vi "Example-血氧仪.vi"() -> ()   [LabVIEW 2018]
uses:
  17504645-33d6-4640-8c4b-92a03107a571.vi
  d24536d2-1b2e-48eb-9735-a10c89dc3041.vi
  40ac2d0d-2d52-431a-8f5c-900a3948c8a2.vi
panel:
  in  "Voltage(V)":dbl=3.3 format="%#_13g"
  in  "Frequency(Hz)":i32(ring)=400 items=["1"=1, "10"=10, "40"=40, "100"=100, "400"=400, "1000"=1000, "4000"=4000, "10000"=10000, "40000"=40000, "100000"=100000, "400000"=400000, "1000000"=1000000, "4000000"=4000000, "10000000"=10000000]
  in  "停止":bool
  in  "addr":u8=87 format="%.0x"
  out "数值":i32
  out "波形图表":cluster{u32, u32}(graph)
  out "SerialNumber":string
  out "rxcount out":i32
  out "rgRX":u8[](array[numeric])
  in  "Tx data":u8[][](array[numeric])=[[9, 64], [2, 12], [3, 0], [4, 0], [5, 0], [6, 0], [8, 15], [9, 3], [10, 39], [12, 50], [13, 50], [16, 127]] format="%.0x"
  in  "SDA IO(0~15)":i32=1
  in  "SCL IO(0~15)":i32
  out "returns":i32[](array[numeric])
  out "error out":errorcluster caption="错误输出"
  in  "error in (no error)":errorcluster caption="错误输入（无错误）"
  out "ftHandle out":u64=363562184
  in  "设备索引":i32
  # "72 75"
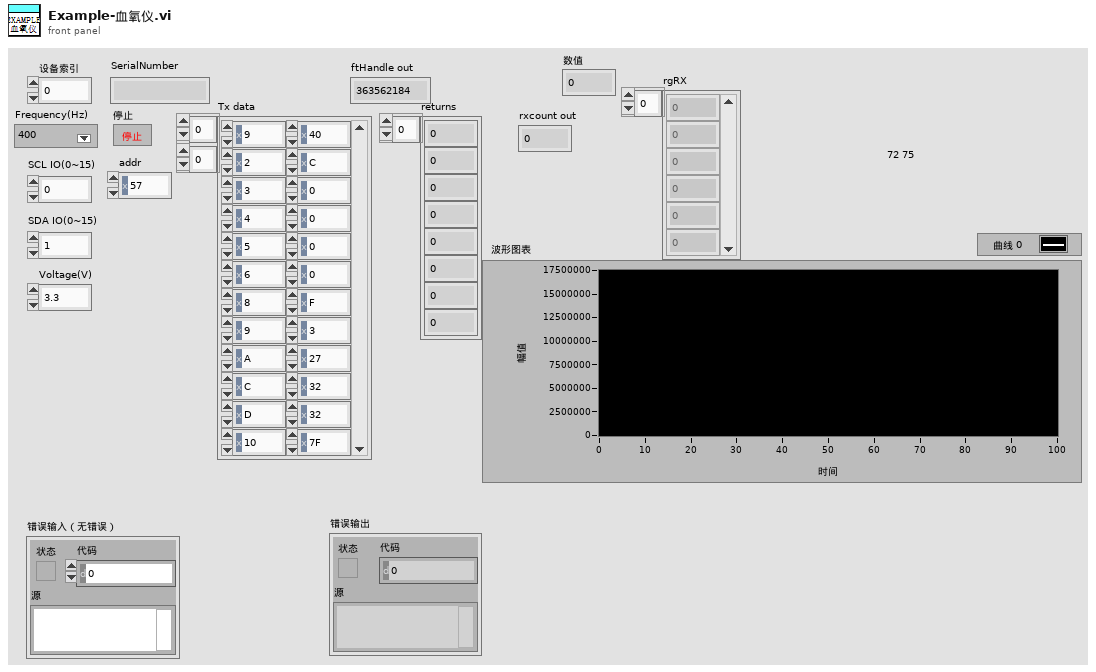
[diagram p1: front panel]
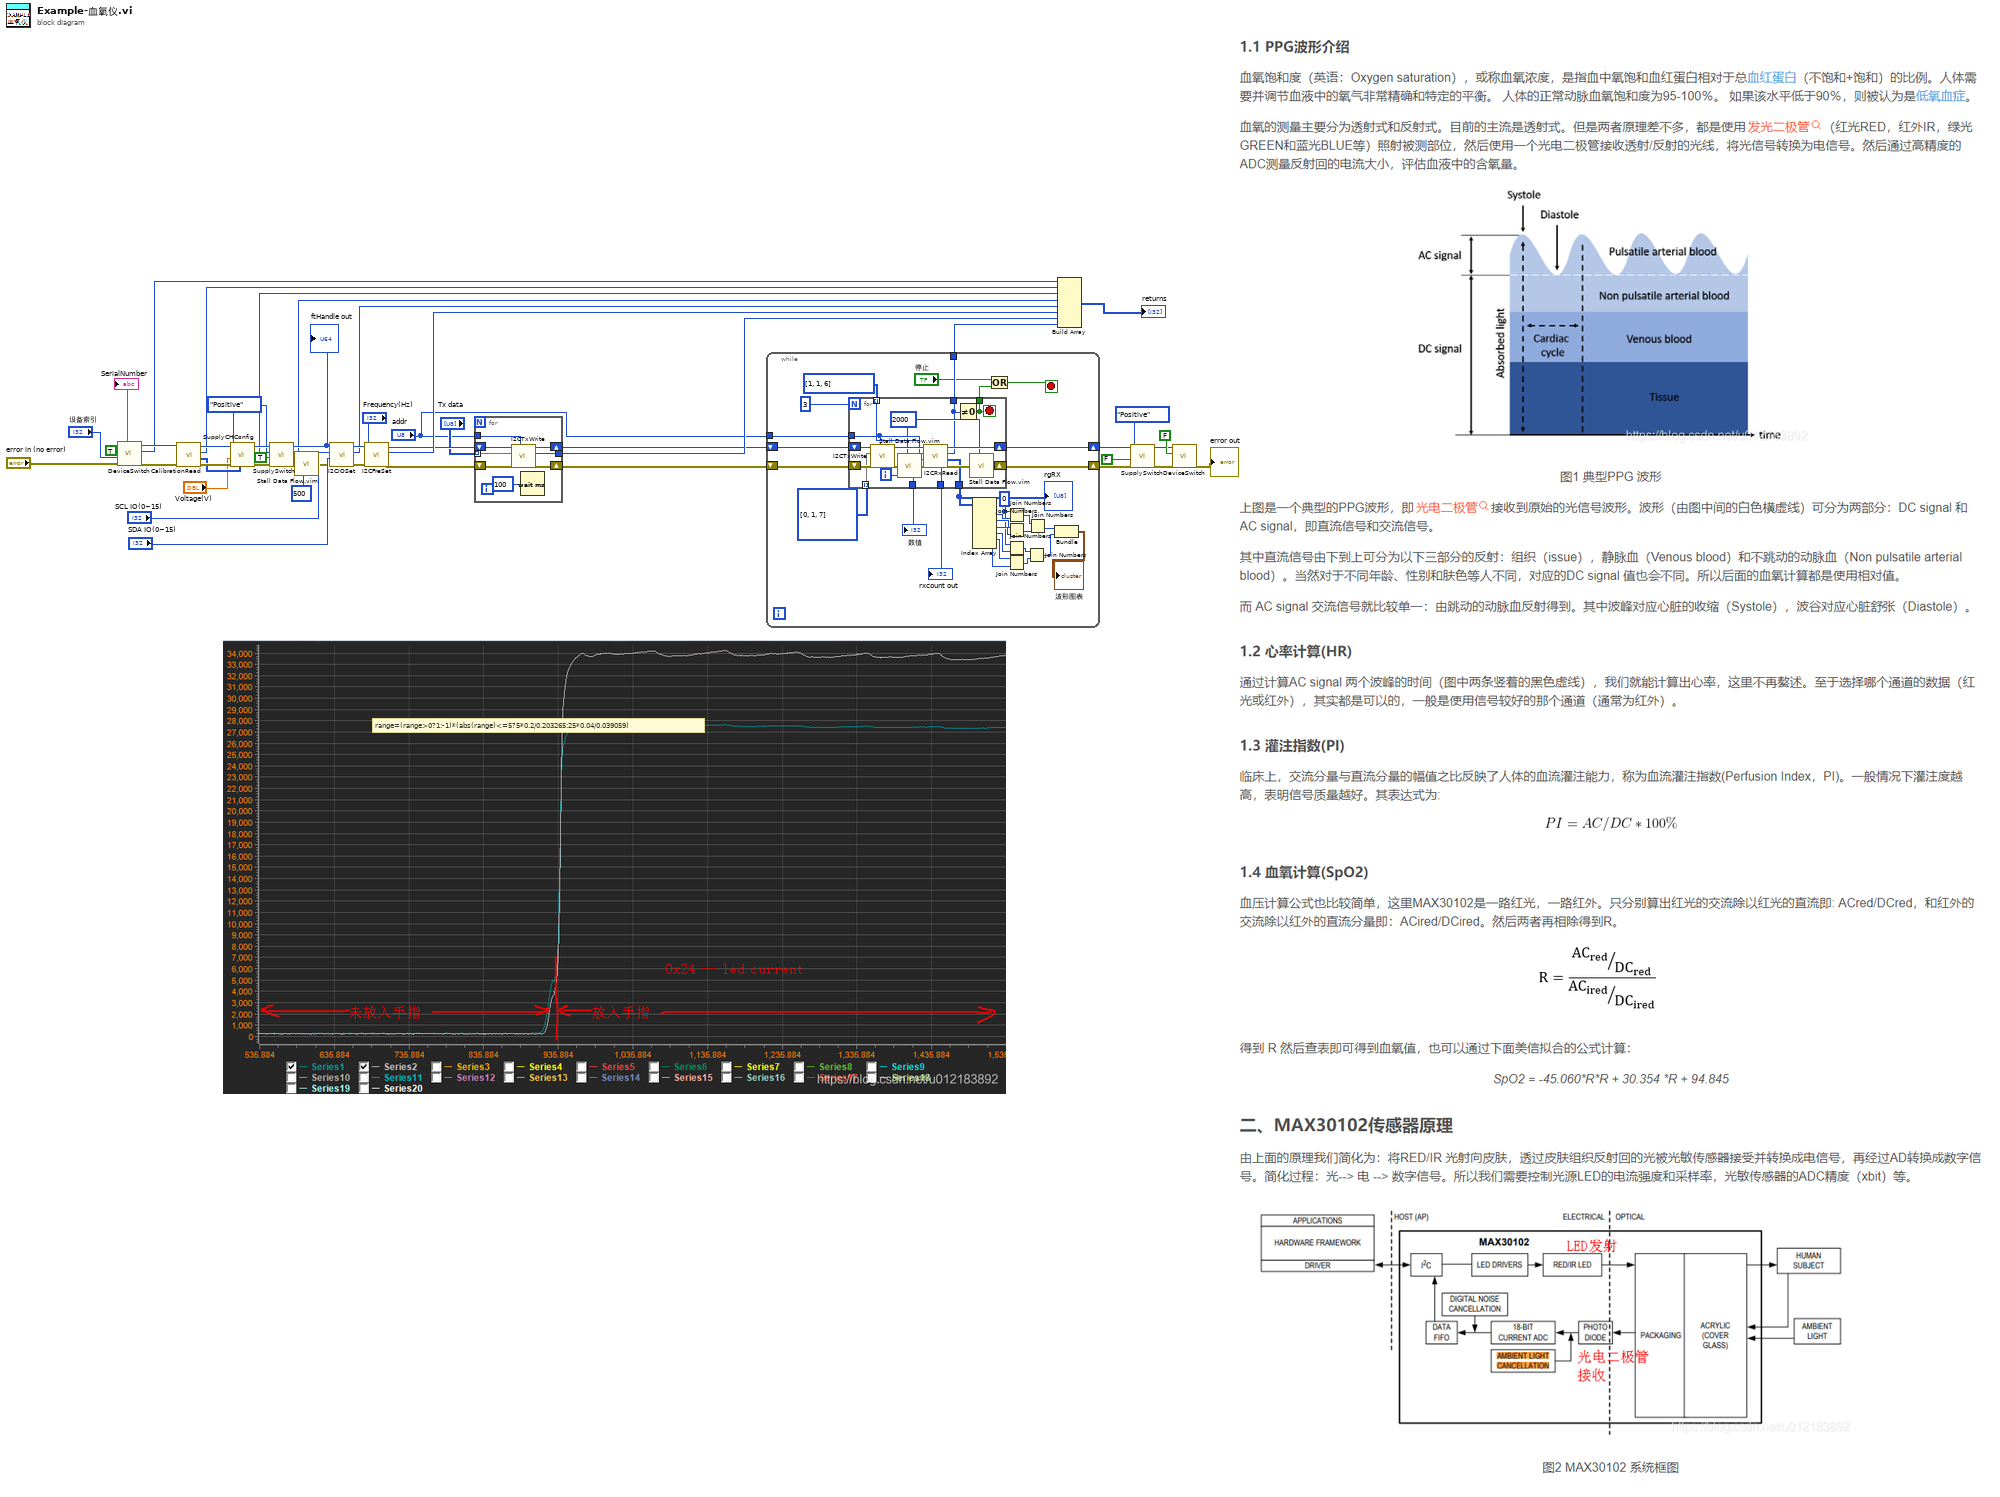
[diagram p0: block diagram]
diagram:
  w24 = enum16{"Positive", "Negative"}."Positive" ("CH")
  # "range=(range>0?1:-1)*(abs(range)<=5?5*0.2/0.203265:25*0.04/0.039059)"
  n1 = call "DeviceSwitch.vi"("error in (no error)"="error in (no error)", "Device Index"="设备索引", "Open"=TRUE) -> ("error out"=w19:errorcluster, "function return"=w15:i32, "handle out"=w18:u64, "SerialNumber"=→"SerialNumber":string)  [unwired: 4 in, 1 out]
  n2 = call "CalibrationRead.vi"("handle"=w18, "error in (no error)"=w19) -> ("handle out"=w21:u64, "function return"=w14:i32, "CalArray"=w20:u8[], "error out"=w22:errorcluster)  [unwired: 5 in]
  n3 = call "SupplyCHConfig.vi"("CalArray"=w20, "error in (no error)"=w22, "Voltage(V)"="Voltage(V)", "CH"=w24, "handle"=w21) -> ("error out"=w25:errorcluster, "function return"=w13:i32, "handle out"=w26:u64)  [unwired: 3 in, 1 out]
  n4 = call "SupplySwitch.vi"("error in (no error)"=w25, "Output"=TRUE, "CH"=w24, "handle"=w26) -> ("error out"=w16:errorcluster, "function return"=w12:i32, "handle out"=w17:u64)  [unwired: 5 in]
  "ftHandle out" <- w17
  n5 = call "Stall Data Flow.vim"("value in"=w16, "milliseconds to wait"=u32 500) -> ("value out"=w4:errorcluster)  [unwired: 1 out]
  n6 = call "I2CIOSet.vi"("error in (no error)"=w4, "SDA IO(0~15)"="SDA IO(0~15)", "SCL IO(0~15)"="SCL IO(0~15)", "handle"=w17) -> ("error out"=w40:errorcluster, "function return"=w36:i32, "handle out"=w37:u64)  [unwired: 5 in]
  n7 = call "I2CFreSet.vi"("error in (no error)"=w40, "Frequency(Hz)"="Frequency(Hz)", "handle"=w37) -> ("error out"=w31:errorcluster, "function return"=w35:i32, "handle out"=w34:u64)  [unwired: 6 in]
  n8 = for {
    tunnel: "Tx data" -> [w48] mode=indexing
    tunnel: [w50] -> w30
    tunnel: "addr" -> [w49]
    shift-right: [w51] -> w2
    shift-left: w34 -> [w54]
    shift-right: [w53] -> w32
    shift-left: w31 -> [w52]
    n9 = call "I2CTxWrite.vi"("addr"=w49, "error in (no error)"=w52, "data"=w48, "handle"=w54) -> ("error out"=w53:errorcluster, "function return"=w50:i32, "handle out"=w51:u64)  [unwired: 5 in]
    n10 = Wait (ms)(milliseconds to wait=u32 100 ("等待时间（毫秒）")) -> ()  [unwired: 1 out]
  }
  n11 = while {
    tunnel: [w79] -> w29
    tunnel: "addr" -> [w75]
    shift-right: [w82] -> w10
    shift-left: w32 -> [w83]
    shift-right: [w81] -> w8
    shift-left: w2 -> [w80]
    stop <- w65 stop-if-true
    w58 = u8 0 ("hi")
    n12 = for {
      N: 3 -> [_]
      tunnel: [w85] -> w79
      tunnel: [w98] -> w73
      tunnel: [w97] -> w78
      shift-right: [w87] -> w82
      shift-left: w83 -> [w94]
      shift-right: [w99] -> w81
      shift-left: w80 -> [w93]
      tunnel: [w96] -> w76
      tunnel: w75 -> [w90]
      tunnel: i32[] [1, 1, 6] -> [w91] mode=indexing
      tunnel: u8[][] [[0], [1], [7]] ("length") -> [w89] mode=indexing
      tunnel: [w84] -> w56
      i -> [w96]
      stop <- w84 stop-if-true
      w86 = u32 2000 ("milliseconds to wait")
      n13 = call "I2CTxWrite.vi"("addr"=w90, "error in (no error)"=w94, "data"=w89, "handle"=w93) -> ("error out"=w95:errorcluster, "handle out"=w92:u64)  [unwired: 5 in, 1 out]
      n14 = call "Stall Data Flow.vim"("value in"=w95, "milliseconds to wait"=w86) -> ("value out"=w88:errorcluster)  [unwired: 1 out]
      n15 = call "I2CRxRead.vi"("error in (no error)"=w88, "addr"=w90, "length"=w91, "handle"=w92) -> ("error out"=w100:errorcluster, "rgRX"=w98:u8[], "function return"=w85:i32, "handle out"=w99:u64, "rxcount out"=w97:i32)  [unwired: 3 in]
      n16 = Not Equal To 0?(x=w85) -> (x != 0?=w84:bool)
      n17 = call "Stall Data Flow.vim"("value in"=w100, "milliseconds to wait"=w86) -> ("value out"=w87:errorcluster)  [unwired: 1 out]
    }
    "rgRX" <- w73
    "rxcount out" <- w78
    "数值" <- w76
    n18 = Index Array(array=w73) -> (element #1=w64:u8, element #2=w63:u8, element #3=w62:u8, element #4=w61:u8, element #5=w60:u8, element #6=w59:u8)  [unwired: 6 in]
    n19 = Or(x="停止", y=w56) -> (x .or. y?=w65:bool)
    n20 = Join Numbers(hi=w58, lo=w64) -> ((hi.lo)=w72:u16)
    n21 = Join Numbers(hi=w63, lo=w62) -> ((hi.lo)=w71:u16)
    n22 = Join Numbers(hi=w60, lo=w59) -> ((hi.lo)=w69:u16)
    n23 = Join Numbers(hi=w58, lo=w61) -> ((hi.lo)=w70:u16)
    n24 = Join Numbers(hi=w70, lo=w69) -> ((hi.lo)=w67:u32)
    n25 = Join Numbers(hi=w72, lo=w71) -> ((hi.lo)=w68:u32)
    n26 = Bundle(w68, w67) -> (→"波形图表":cluster{u32, u32})  [unwired: 1 in]
  }
  n27 = Build Array(w15, w14, w13, w12, w36, w35, w30, w29) -> (→"returns":i32[])
  n28 = call "SupplySwitch.vi"("error in (no error)"=w10, "Output"=FALSE, "CH"=enum16{"Positive", "Negative"}."Positive", "handle"=w8) -> ("error out"=w9:errorcluster, "handle out"=w7:u64)  [unwired: 5 in, 1 out]
  n29 = call "DeviceSwitch.vi"("error in (no error)"=w9, "Open"=FALSE, "handle"=w7) -> ("error out"=→"error out":errorcluster)  [unwired: 4 in, 4 out]
